vi "Run SPARC 3.1.vi"(8 "error in (no error)":errorcluster, 11 "Data Cluster In":T1={"Selected File"=path "", "Full Text File"=[], "Data Array"=[], "Times Array"=[], "Sensor Array"=[], "Subset Array"=[], "Smoothness Values"=[], "Sensor Select 1"=refnum, "Sensor Select 2"=refnum, "Sensor Select 3"=refnum, "Sensor Select 4"=refnum, "Start Times"=[], "End Times"=[], "Cursor List"=[{"Name"="Event Marker          ", "Color"=16777200, "Style"=0, "Point Style"=0, "Name Visible"=FALSE, "Allow Drag"=FALSE, "Cursor Mode"=0, "Plot"=0, "Index"=0, "Position"={"X"=4.0, "Y"=1.0}, "X Scale"=0, "Y Scale"=0, "Watch Plots"=[], "Watch All Plots"=FALSE, "Plot Area"=0, "Label Offset"={"X"=-50.0, "Y"=150.0}}, {"Name"="Upper Sensor", "Color"=13816500, "Style"=6, "Point Style"=0, "Name Visible"=FALSE, "Allow Drag"=FALSE, "Cursor Mode"=0, "Plot"=0, "Index"=0, "Position"={"X"=-1.0, "Y"=5.0}, "X Scale"=0, "Y Scale"=0, "Watch Plots"=[], "Watch All Plots"=FALSE, "Plot Area"=0, "Label Offset"={"X"=0.0, "Y"=0.0}}, {"Name"="Lower Sensor", "Color"=13816500, "Style"=6, "Point Style"=0, "Name Visible"=FALSE, "Allow Drag"=FALSE, "Cursor Mode"=0, "Plot"=0, "Index"=0, "Position"={"X"=-1.0, "Y"=30.0}, "X Scale"=0, "Y Scale"=0, "Watch Plots"=[], "Watch All Plots"=FALSE, "Plot Area"=0, "Label Offset"={"X"=0.0, "Y"=0.0}}], "Listbox 1"=refnum, "Listbox 2"=refnum, "Listbox 3"=refnum, "Listbox 4"=refnum, "Labels"=["Why", "is", "this", "still", "not", "built", "into", "Labview?", "This", "is", "shameful."], "Event Array"=[], "Event Names"=[], "Event Times"=[], "Save Plot Button"=refnum, "Sensor Plot Refs"=[], "Selected Event (Title)"="", "Upper Cursor"=0.0, "Lower Cursor"=0.0, "Z Max"=0.0, "Z Min"=0.0}) -> (0 "error out":errorcluster, 3 "Data Cluster Out":T1={"Selected File"=path "", "Full Text File"=[], "Data Array"=[], "Times Array"=[], "Sensor Array"=[], "Subset Array"=[], "Smoothness Values"=[], "Sensor Select 1"=refnum, "Sensor Select 2"=refnum, "Sensor Select 3"=refnum, "Sensor Select 4"=refnum, "Start Times"=[], "End Times"=[], "Cursor List"=[{"Name"="Event Marker          ", "Color"=16777200, "Style"=0, "Point Style"=0, "Name Visible"=FALSE, "Allow Drag"=FALSE, "Cursor Mode"=0, "Plot"=0, "Index"=0, "Position"={"X"=4.0, "Y"=1.0}, "X Scale"=0, "Y Scale"=0, "Watch Plots"=[], "Watch All Plots"=FALSE, "Plot Area"=0, "Label Offset"={"X"=-50.0, "Y"=150.0}}, {"Name"="Upper Sensor", "Color"=13816500, "Style"=6, "Point Style"=0, "Name Visible"=FALSE, "Allow Drag"=FALSE, "Cursor Mode"=0, "Plot"=0, "Index"=0, "Position"={"X"=-1.0, "Y"=5.0}, "X Scale"=0, "Y Scale"=0, "Watch Plots"=[], "Watch All Plots"=FALSE, "Plot Area"=0, "Label Offset"={"X"=0.0, "Y"=0.0}}, {"Name"="Lower Sensor", "Color"=13816500, "Style"=6, "Point Style"=0, "Name Visible"=FALSE, "Allow Drag"=FALSE, "Cursor Mode"=0, "Plot"=0, "Index"=0, "Position"={"X"=-1.0, "Y"=30.0}, "X Scale"=0, "Y Scale"=0, "Watch Plots"=[], "Watch All Plots"=FALSE, "Plot Area"=0, "Label Offset"={"X"=0.0, "Y"=0.0}}], "Listbox 1"=refnum, "Listbox 2"=refnum, "Listbox 3"=refnum, "Listbox 4"=refnum, "Labels"=["Why", "is", "this", "still", "not", "built", "into", "Labview?", "This", "is", "shameful."], "Event Array"=[], "Event Names"=[], "Event Times"=[], "Save Plot Button"=refnum, "Sensor Plot Refs"=[], "Selected Event (Title)"="", "Upper Cursor"=0.0, "Lower Cursor"=0.0, "Z Max"=0.0, "Z Min"=0.0})   [LabVIEW 2021]
uses:
  Controls/DataCluster.ctl
  <vilib>/Utility/miscctls.llb/LVCursorListTypeDef.ctl
  Controls/SPARC Analysis States.ctl
  <userlib>/_OpenG.lib/file/file.llb/File Exists - Scalar__ogtk.vi
panel:
  out "SPARC Plot":picture
  out "Selected Segment":dbl[][](graph)
  out "Saving":bool
  out "Analyzing":bool
  out "Segmenting":bool
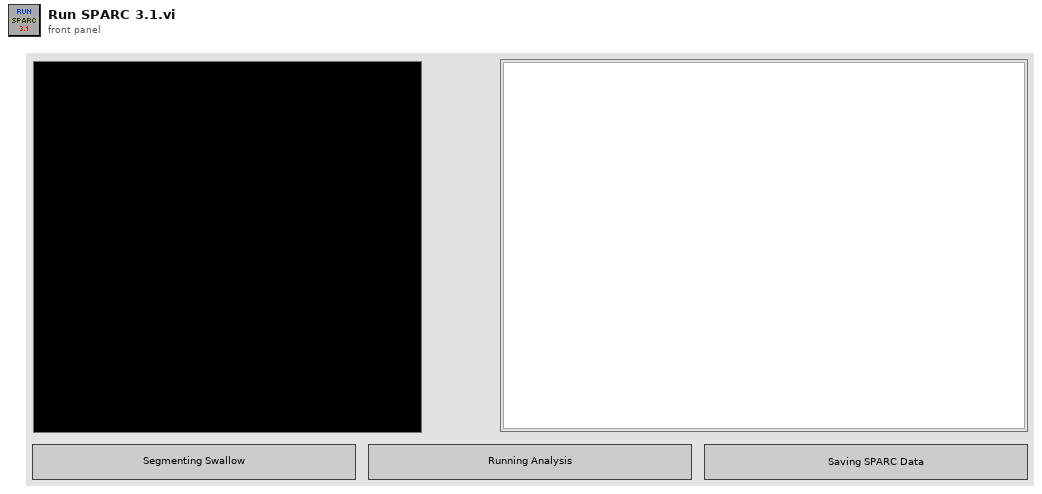
[diagram p1: front panel]
types:
  T1 = typedef "DataCluster.ctl" = cluster{"Selected File":path, "Full Text File":string[][], "Data Array":dbl[][], "Times Array":dbl[], "Sensor Array":dbl[], "Subset Array":dbl[][], "Smoothness Values":dbl[], "Sensor Select 1":refnum<vi>, "Sensor Select 2":refnum<vi>, "Sensor Select 3":refnum<vi>, "Sensor Select 4":refnum<vi>, "Start Times":dbl[], "End Times":dbl[], "Cursor List":T2, "Listbox 1":refnum<vi>, "Listbox 2":refnum<vi>, "Listbox 3":refnum<vi>, "Listbox 4":refnum<vi>, "Labels":string[], "Event Array":dbl[][], "Event Names":string[], "Event Times":dbl[], "Save Plot Button":refnum<vi>, "Sensor Plot Refs":refnum<vi>[], "Selected Event (Title)":string, "Upper Cursor":dbl, "Lower Cursor":dbl, "Z Max":dbl, "Z Min":dbl}
  T2 = typedef "LVCursorListTypeDef.ctl" = cluster{"Name":string, "Color":u32, "Style":u8, "Point Style":u8, "Name Visible":bool, "Allow Drag":bool, "Cursor Mode":u32, "Plot":i32, "Index":i32, "Position":cluster{"X":dbl, "Y":dbl}, "X Scale":u32, "Y Scale":u32, "Watch Plots":i32[], "Watch All Plots":bool, "Plot Area":i32, "Label Offset":cluster{"X":dbl, "Y":dbl}}[]
  T3 = enum16{"open", "replace", "create", "open or create", "replace or create", "replace or create with confirmation"}
  T4 = typedef "SPARC Analysis States.ctl" = enum16{"Segment", "Analyze", "Save"}
  T5 = cluster{"Cursor List[0]":cluster{"Name":string, "Color":u32, "Style":u8, "Point Style":u8, "Name Visible":bool, "Allow Drag":bool, "Cursor Mode":u32, "Plot":i32, "Index":i32, "Position":cluster{"X":dbl, "Y":dbl}, "X Scale":u32, "Y Scale":u32, "Watch Plots":i32[], "Watch All Plots":bool, "Plot Area":i32, "Label Offset":cluster{"X":dbl, "Y":dbl}}, "Cursor List[1]":cluster{"Name":string, "Color":u32, "Style":u8, "Point Style":u8, "Name Visible":bool, "Allow Drag":bool, "Cursor Mode":u32, "Plot":i32, "Index":i32, "Position":cluster{"X":dbl, "Y":dbl}, "X Scale":u32, "Y Scale":u32, "Watch Plots":i32[], "Watch All Plots":bool, "Plot Area":i32, "Label Offset":cluster{"X":dbl, "Y":dbl}}, "Cursor List[2]":cluster{"Name":string, "Color":u32, "Style":u8, "Point Style":u8, "Name Visible":bool, "Allow Drag":bool, "Cursor Mode":u32, "Plot":i32, "Index":i32, "Position":cluster{"X":dbl, "Y":dbl}, "X Scale":u32, "Y Scale":u32, "Watch Plots":i32[], "Watch All Plots":bool, "Plot Area":i32, "Label Offset":cluster{"X":dbl, "Y":dbl}}, "Cursor List[3]":cluster{"Name":string, "Color":u32, "Style":u8, "Point Style":u8, "Name Visible":bool, "Allow Drag":bool, "Cursor Mode":u32, "Plot":i32, "Index":i32, "Position":cluster{"X":dbl, "Y":dbl}, "X Scale":u32, "Y Scale":u32, "Watch Plots":i32[], "Watch All Plots":bool, "Plot Area":i32, "Label Offset":cluster{"X":dbl, "Y":dbl}}, "Cursor List[4]":cluster{"Name":string, "Color":u32, "Style":u8, "Point Style":u8, "Name Visible":bool, "Allow Drag":bool, "Cursor Mode":u32, "Plot":i32, "Index":i32, "Position":cluster{"X":dbl, "Y":dbl}, "X Scale":u32, "Y Scale":u32, "Watch Plots":i32[], "Watch All Plots":bool, "Plot Area":i32, "Label Offset":cluster{"X":dbl, "Y":dbl}}, "Cursor List[5]":cluster{"Name":string, "Color":u32, "Style":u8, "Point Style":u8, "Name Visible":bool, "Allow Drag":bool, "Cursor Mode":u32, "Plot":i32, "Index":i32, "Position":cluster{"X":dbl, "Y":dbl}, "X Scale":u32, "Y Scale":u32, "Watch Plots":i32[], "Watch All Plots":bool, "Plot Area":i32, "Label Offset":cluster{"X":dbl, "Y":dbl}}, "Cursor List[6]":cluster{"Name":string, "Color":u32, "Style":u8, "Point Style":u8, "Name Visible":bool, "Allow Drag":bool, "Cursor Mode":u32, "Plot":i32, "Index":i32, "Position":cluster{"X":dbl, "Y":dbl}, "X Scale":u32, "Y Scale":u32, "Watch Plots":i32[], "Watch All Plots":bool, "Plot Area":i32, "Label Offset":cluster{"X":dbl, "Y":dbl}}, "Cursor List[7]":cluster{"Name":string, "Color":u32, "Style":u8, "Point Style":u8, "Name Visible":bool, "Allow Drag":bool, "Cursor Mode":u32, "Plot":i32, "Index":i32, "Position":cluster{"X":dbl, "Y":dbl}, "X Scale":u32, "Y Scale":u32, "Watch Plots":i32[], "Watch All Plots":bool, "Plot Area":i32, "Label Offset":cluster{"X":dbl, "Y":dbl}}, "Cursor List[8]":cluster{"Name":string, "Color":u32, "Style":u8, "Point Style":u8, "Name Visible":bool, "Allow Drag":bool, "Cursor Mode":u32, "Plot":i32, "Index":i32, "Position":cluster{"X":dbl, "Y":dbl}, "X Scale":u32, "Y Scale":u32, "Watch Plots":i32[], "Watch All Plots":bool, "Plot Area":i32, "Label Offset":cluster{"X":dbl, "Y":dbl}}}
  T6 = cluster{"Name":string, "Color":u32, "Style":u8, "Point Style":u8, "Name Visible":bool, "Allow Drag":bool, "Cursor Mode":u32, "Plot":i32, "Index":i32, "Position":cluster{"X":dbl, "Y":dbl}, "X Scale":u32, "Y Scale":u32, "Watch Plots":i32[], "Watch All Plots":bool, "Plot Area":i32, "Label Offset":cluster{"X":dbl, "Y":dbl}}[]
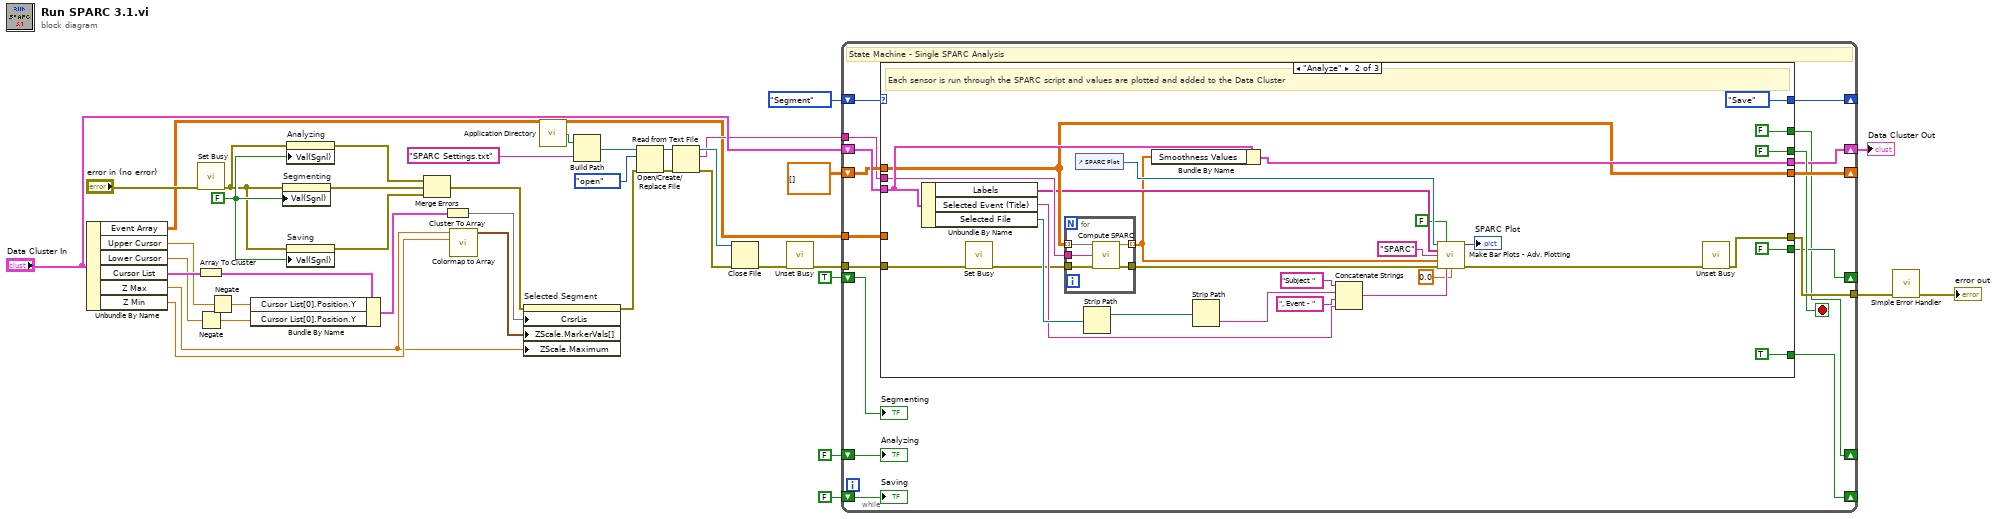
[diagram p0: block diagram]
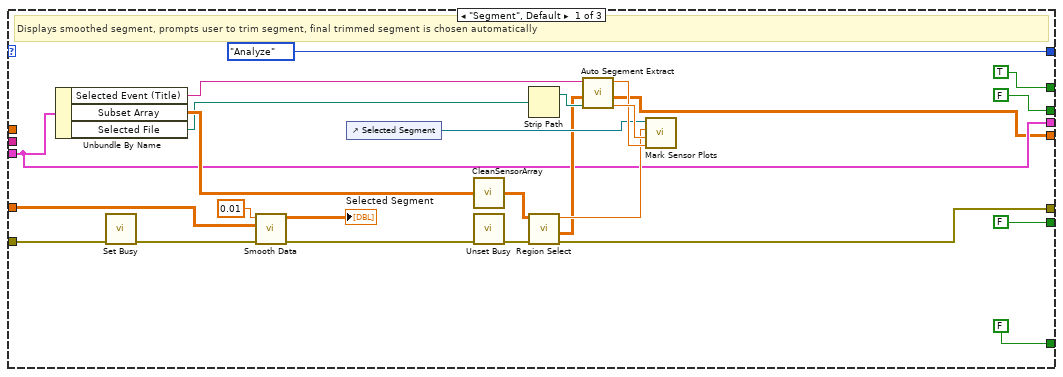
[diagram p2: hidden frame]
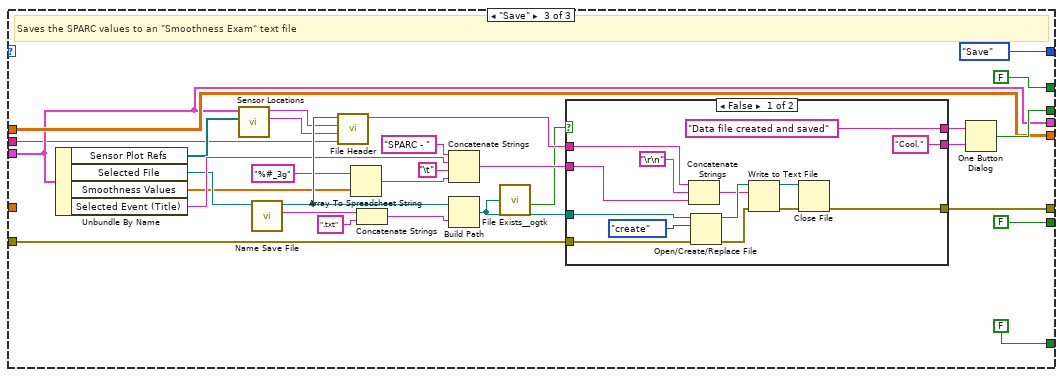
[diagram p3: hidden frame]
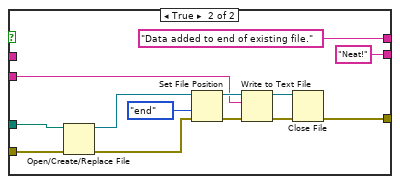
[diagram p4: hidden frame]
diagram:
  w9 = FALSE ("Value (Signaling)")
  n1 = Unbundle By Name("Data Cluster In") -> ("Event Array"=w10:dbl[][], "Upper Cursor"=w35:dbl, "Lower Cursor"=w34:dbl, "Cursor List"=w40:T2, "Z Max"=w21:dbl, "Z Min"=w22:dbl)
  n2 = Array To Cluster(array=w40) -> (cluster=w39:T5)
  n3 = call <vilib>:"Set Busy.vi"("error in (no error)"="error in (no error)") -> ("error out"=w3:errorcluster)  [unwired: 9 in, 1 out]
  n4 = Negate(x=w34) -> (-x=w36:dbl)
  n5 = Negate(x=w35) -> (-x=w37:dbl)
  n6 = Bundle By Name(cluster=w39, "Cursor List[0].Position.Y"=w37, "Cursor List[0].Position.Y"=w36) -> (w38:T5)
  n7 = property on="Segmenting" class="Bool (strict)"(error in=w3, "Val(Sgnl)"=w9) -> (error out=w7:errorcluster)  [unwired: 1 in, 1 out]
  n8 = property on="Analyzing" class="Bool (strict)"(error in=w3, "Val(Sgnl)"=w9) -> (error out=w8:errorcluster)  [unwired: 1 in, 1 out]
  n9 = property on="Saving" class="Bool (strict)"(error in=w3, "Val(Sgnl)"=w9) -> (error out=w6:errorcluster)  [unwired: 1 in, 1 out]
  n10 = Merge Errors(w8, w7, w6) -> (w4:errorcluster)
  n11 = Cluster To Array(cluster=w38) -> (array=w26:T6)
  n12 = call "Colormap to Array.vi"("Min Pressure"=w22, "Max Pressure"=w21) -> ("Z Scale.Marker Values[]"=w25:cluster{dbl, u32}[])  [unwired: 9 in]
  n13 = property on="Selected Segment" class="IntGraph (strict)"(error in=w4, "CrsrLis"=w26, "ZScale.MarkerVals[]"=w25, "ZScale.Maximum"=w21) -> (error out=w5:errorcluster)  [unwired: 1 in, 1 out]
  n14 = call <vilib>:"Application Directory.vi"() -> ("Application Directory"=w20:path)
  n15 = Build Path(base path=w20, name or relative path="SPARC Settings.txt") -> (appended path=w19:path)
  n16 = Open/Create/Replace File(file path (use dialog)=w19, error in=w5, operation (0:open)=T3."open") -> (refnum out=w18:refnum<file>, error out=w16:errorcluster)  [unwired: 3 in, 1 out]
  n17 = Read from Text File(file (use dialog)=w18, error in=w16) -> (refnum out=w17:refnum<file>, text=w13:string, error out=w15:errorcluster)  [unwired: 2 in, 1 out]
  n18 = Close File(refnum=w17, error in=w15) -> (error out=w11:errorcluster)  [unwired: 1 out]
  n19 = call <vilib>:"Unset Busy.vi"("error in (no error)"=w11) -> ("error out"=w31:errorcluster)  [unwired: 10 in]
  n20 = while {
    tunnel: w31 -> [w55]
    tunnel: [w56] -> w2
    shift-right: [w57] -> _
    shift-left: dbl[][] [] ("Trimmed Segment") -> [w53]
    shift-right: [w51] -> w23
    shift-left: "Data Cluster In" -> [w54]
    shift-right: [w47] -> _
    shift-left: TRUE -> [w50]
    shift-right: [w46] -> _
    shift-left: FALSE -> [w49]
    shift-right: [w45] -> _
    shift-left: FALSE -> [w48]
    shift-right: [w43] -> _
    shift-left: SPARC_Analysis_States."Segment" -> [w44]
    tunnel: w13 -> [w42]
    tunnel: w10 -> [w41]
    stop <- w52 stop-if-true
    # "State Machine - Single SPARC Analysis"
    n21 = case shown="\"Analyze\"" w44 {
      tunnel: w55 -> [w61 w97 w126]
      tunnel: w54 -> [w71 w101 w122]
      tunnel: [w58 w98 w123] -> w57
      tunnel: [w59 w100 w124] -> w56
      tunnel: w53 -> [_ w98 w123]
      tunnel: [w71 w102 w122] -> w51
      tunnel: [FALSE ("true") FALSE ("true") w125] -> w52
      tunnel: [FALSE FALSE FALSE] -> w47
      tunnel: [TRUE FALSE FALSE] -> w46
      tunnel: [FALSE TRUE FALSE] -> w45
      tunnel: [SPARC_Analysis_States."Analyze" SPARC_Analysis_States."Save" SPARC_Analysis_States."Save"] -> w43
      tunnel: w42 -> [_ w91 w117]
      tunnel: w41 -> [w65 _ _]
      frame "Segment", Default {
        # "Displays smoothed segment, prompts user to trim segment, final trimmed segment is chosen automatically"
        n22 = Unbundle By Name(w71) -> ("Selected Event (Title)"=w76:string, "Subset Array"=w74:dbl[][], "Selected File"=w73:path)
        n23 = call <vilib>:"Set Busy.vi"("error in (no error)"=w61) -> ("error out"=w63:errorcluster)  [unwired: 9 in, 1 out]
        n24 = call "Smooth Data.vi"("error in (no error)"=w63, "Data Array"=w65, "dt"=0.01) -> ("error out"=w62:errorcluster, "Resampled Array"=→"Selected Segment":dbl[][])  [unwired: 7 in]
        n25 = control-ref of="Selected Segment"() -> (w79:refnum<vi>)
        n26 = call "CleanSensorArray.vi"("Sensor Data Array"=w74) -> ("Clean Array"=w75:dbl[][])  [unwired: 4 in]
        n27 = call <vilib>:"Unset Busy.vi"("error in (no error)"=w62) -> ("error out"=w60:errorcluster)  [unwired: 10 in]
        n28 = Strip Path(path=w73) -> (stripped path=w78:path)  [unwired: 1 out]
        n29 = call "Region Select.vi"("Error In"=w60, "Sensor Data Array"=w75) -> ("Error Out"=w59:errorcluster, "Trimmed Event"=w77:dbl[][], "Segement Start"=w80:dbl)  [unwired: 7 in]
        n30 = call "Auto Segement Extract.vi"("Save Path"=w78, "Sensor Data Array"=w77, "Title"=w76) -> ("End"=w82:dbl, "Trimmed Segment"=w58:dbl[][], "Start"=w81:dbl)  [unwired: 1 in, 1 out]
        n31 = call "Mark Sensor Plots.vi"("Segment Select Ref"=w79, "Segement Start"=w80, "End"=w82, "Start"=w81) -> ()  [unwired: 7 in]
      }
      frame "Analyze" {
        # "Each sensor is run through the SPARC script and values are plotted and added to the Data Cluster"
        n32 = Unbundle By Name(w101) -> ("Labels"=w89:string[], "Selected Event (Title)"=w88:string, "Selected File"=w90:path)
        n33 = call <vilib>:"Set Busy.vi"("error in (no error)"=w97) -> ("error out"=w85:errorcluster)  [unwired: 9 in, 1 out]
        n34 = for {
          tunnel: w98 -> [w113] mode=indexing
          tunnel: [w115] -> w107
          tunnel: [w114] -> w86 mode=indexing
          tunnel: w91 -> [w112]
          tunnel: w85 -> [w111]
          n35 = call "Compute SPARC.vi"("Pressure Array"=w113, "Settings"=w112, "error in"=w111) -> ("SPARC"=w114:dbl, "error out"=w115:errorcluster)  [unwired: 11 in]
        }
        n36 = control-ref of="SPARC Plot"() -> (w106:refnum<vi>)
        n37 = Strip Path(path=w90) -> (stripped path=w87:path)  [unwired: 1 out]
        n38 = Bundle By Name(cluster=w101, "Smoothness Values"=w86) -> (w102:T1)
        n39 = Strip Path(path=w87) -> (name=w109:string)  [unwired: 1 out]
        n40 = Concatenate Strings("Subject " ("string"), w109, ", Event - " ("string"), w88) -> (w108:string)
        n41 = call "Make Bar Plots - Adv. Plotting.vi"("Picture in"=w106, "Save Plot?"=FALSE, "Labels"=w89, "Legend Title"="SPARC", "SPARC"=w86, "error in (no error)"=w107, "Title"=w108, "Y Min"=0.0) -> ("Picture"=→"SPARC Plot":picture, "error out"=w110:errorcluster)  [unwired: 6 in]
        n42 = call <vilib>:"Unset Busy.vi"("error in (no error)"=w110) -> ("error out"=w100:errorcluster)  [unwired: 10 in]
      }
      frame "Save" {
        # "Saves the SPARC values to an \"Smoothness Exam\" text file"
        n43 = Unbundle By Name(w122) -> ("Sensor Plot Refs"=w133:refnum<vi>[], "Selected File"=w132:path, "Smoothness Values"=w116:dbl[], "Selected Event (Title)"=w135:string)
        n44 = call "Sensor Locations.vi"("Ref Array"=w133, "Data Cluster In"=w122) -> ("Sensors"=w138:string, "Locations"=w137:string)  [unwired: 8 in]
        n45 = call "Name Save File.vi"("Selected File"=w132) -> ("Name"=w140:string, "stripped path"=w141:path)  [unwired: 9 in]
        n46 = call "File Header.vi"("Settings"=w117, "Sensors"=w138, "Locations"=w137, "Stripped Path"=w141) -> ("File Header"=w139:string)  [unwired: 7 in]
        n47 = Array To Spreadsheet String(array=w116, 3:"%#_3g" ("format string")) -> (spreadsheet string=w136:string)  [unwired: 1 in]
        n48 = Concatenate Strings(w140, ".txt" ("string")) -> (w131:string)
        n49 = Concatenate Strings("SPARC - " ("string"), w135, "\t", w136) -> (w144:string)
        n50 = Build Path(base path=w141, name or relative path=w131) -> (appended path=w145:path)
        n51 = call-poly <userlib>:"File Exists__ogtk.vi"("file path"=w145) -> ("exists"=w134:bool)  [unwired: 6 in, 1 out]
        n52 = case shown="False" w134 {
          tunnel: w139 -> [w147 _]
          tunnel: w145 -> [w158 w172]
          tunnel: [w154 w166] -> w124
          tunnel: ["Data file created and saved" "Data added to end of existing file."] -> w142
          tunnel: ["Cool." "Neat!"] -> w143
          tunnel: w144 -> [w148 w161]
          tunnel: w126 -> [w149 w160]
          frame False {
            n53 = Concatenate Strings(w147, "\r\n", w148) -> (w150:string)
            n54 = Open/Create/Replace File(file path (use dialog)=w158, error in=w149, operation (0:open)=T3."create") -> (refnum out=w157:refnum<file>, error out=w156:errorcluster)  [unwired: 3 in, 1 out]
            n55 = Write to Text File(file (use dialog)=w157, text=w150, error in=w156) -> (refnum out=w153:refnum<file>, error out=w155:errorcluster)  [unwired: 1 in, 1 out]
            n56 = Close File(refnum=w153, error in=w155) -> (error out=w154:errorcluster)  [unwired: 1 out]
          }
          frame True {
            n57 = Open/Create/Replace File(file path (use dialog)=w172, error in=w160) -> (refnum out=w170:refnum<file>, error out=w169:errorcluster)  [unwired: 4 in, 1 out]
            n58 = Set File Position(refnum=w170, from (0:start)=enum16{"start", "end", "current"}."end", error in=w169) -> (refnum out=w165:refnum<file>, error out=w168:errorcluster)  [unwired: 1 in]
            n59 = Write to Text File(file (use dialog)=w165, text=w161, error in=w168) -> (refnum out=w164:refnum<file>, error out=w167:errorcluster)  [unwired: 1 in, 1 out]
            n60 = Close File(refnum=w164, error in=w167) -> (error out=w166:errorcluster)  [unwired: 1 out]
          }
        }
        n61 = One Button Dialog(message=w142, button name ("OK")=w143) -> (true=w125:bool)
      }
    }
    "Saving" <- w48
    "Analyzing" <- w49
    "Segmenting" <- w50
  }
  "Data Cluster Out" <- w23
  n62 = call <vilib>:"Simple Error Handler.vi"("error in (no error)"=w2) -> ("error out"=→"error out":errorcluster)  [unwired: 4 in, 4 out]
